vi "BusTapeAlignment.vi"() -> ()   [LabVIEW 2016]
uses:
  <vilib>/vision/Image Controls.llb/IMAQ Image.ctl
  <vilib>/vision/Measure.llb/Edge Options.ctl
  <vilib>/vision/Measure.llb/Edge Polarity.ctl
  <vilib>/Analysis/6fits.llb/Curve Fitting Criteria.ctl
  <vilib>/vision/NI_Vision_Development_Module.lvlib
  <vilib>/Analysis/NI_AALPro.lvlib
  <vilib>/Analysis/NI_AALBase.lvlib
panel:
  out "Image Frame":dbl[][](array[numeric])
  out "Locations":dbl[][](array[numeric])
  in  "Sample Size":dbl
  out "Output Cluster Array (Top/Bottom)":T1(array[cluster])
  in  "um/pix resolution":dbl=1.5
  in  "Template Path":path=path "D:/Git/StaveAssembly/XYZstage+Camera_CollectedImages/2017-03-03/1_Dots_WorkingDistanceCalibTemplate_z1p0.png"
  in  "Input Images Array":T2[](array[typedef])
  in  "Input Coordinate Array":dbl[][](array[numeric])
  in  "Test?":bool
  out "Bottom errors (um)":dbl[][](array[numeric])
  out "Top errors (um)":dbl[][](array[numeric])
  out "Bottom":cluster{"Bottom":dbl[], "Bottom":dbl[]}[](graph)
  out "Bottom \nResiduals (um)":dbl[](array[numeric])
  out "Top \nResiduals (um)":dbl[](array[numeric])
  out "Top":cluster{"Top":dbl[], "Top":dbl[]}[](graph)
  in  "method":T3 items=["Least Square", "Least Absolute Residual", "Bisquare"]
  out "Bottom":dbl[][](array[numeric])
  out "Top":dbl[][](array[numeric])
  out "Coordinate array for image capture":dbl[][](array[numeric])
  out "Processing Image #":i32
  out "Selected subarray":T2(plugin-control)
  out "Fitted Circle":T4 {"Average SNR (dB)" format="%.2f"; "Average Strength" format="%.2f"; "Roundness (Real-World)" format="%.2f"; "Radius (Real-World)" format="%.2f"; "Center (Real-World)"."Y" format="%.2f"; "Center (Real-World)"."X" format="%.2f"; "Radius (Pixels)" format="%.2f"; "Center (Pixels)"."Y" format="%.2f"; "Center (Pixels)"."X" format="%.2f"}
  in  "Circle ROI Descriptor":T5={"Global Rectangle"=[675, 567, 1751, 1642], "Contours"=[{"ID"=enum."External", "Type"=7, "Coordinates"=[1212, 1104, 190, 250, 0, 0]}]} {"Contours"."Type" items=["No Selection", "Point", "Line", "Rectangle", "Oval", "Polygon", "Freehand Region", "Annulus", "Unused2", "Unused3", "Broken Line", "Freehand Line", "Rotated Rectangle"]}
  in  "Circle Fit Options":T6={"Process"=enum."Get Best Edge", "Step Size"=3.0, "Max Pixel Radius"=3}
  in  "Circle Finding Options":T9={"Search  Direction"=1, "Edge Options"={"Edge Polarity"=2, "Kernel Size"=3, "Width"=3, "Minimum Edge Strength"=10.0, "Interpolation Type"=enum."Bilinear Fixed", "Data Processing Method"=enum."Median"}, "Show Search Area"=TRUE, "Show Search Lines"=TRUE, "Show Edges Found"=TRUE, "Show Result"=TRUE, "Search Area Color"=65280, "Search Lines Color"=255, "Edge Locations Color"=16776960, "Result Color"=65511, "Overlay Group Name"=""} {"Search  Direction" items=["Outside to Inside", "Inside to Outside"]; "Edge Options"."Edge Polarity" items=["All Edges", "Rising Edges", "Falling Edges"]; "Edge Options"."Minimum Edge Strength" format="%.2f"; "Edge Options"."Width" step=2; "Edge Options"."Kernel Size" step=2}
  in  "Pattern Match Settings":T10={"Algorithm"=2, "Number of Matches Requested"=1, "Minimum Match Score"=800.0, "SubPixel Accuracy"=TRUE, "Rotation Angle Ranges"=[], "Show Search Area"=FALSE, "Show Result"=TRUE} {"Rotation Angle Ranges"."End" format="%.1f"; "Rotation Angle Ranges"."Start" format="%.1f"; "Minimum Match Score" min=0 max=1000 format="%.2f"; "Number of Matches Requested" min=1; "Algorithm" items=["All", "Low Discrepancy Sampling", "Grayscale Value Pyramid", "Gradients Pyramid"]}
  out "Template Image":T2
  in  "Coordinate file for image capture":path=path "D:/Git/StaveAssembly/XYZstage+Camera_CollectedImages/2017-03-15/BrendonsFidMarks_dots_2017-03-15-captured.csv"
  out "Review":bool
  out "Search running?":bool
  in  "Stop and delete":bool
  out "Images Array":T2[](array[plugin-control])=["image_442_-22_00"]
  in  "error in":errorcluster
  out "error out":errorcluster
  out "Filenames Array":string[](array[string])=["image_442_-22_110.png", "image_442_-22_137.png", "image_442_-22_192.png", "image_442_-22_222.png", "image_442_-22_26.png", "image_442_-22_56.png"]
  in  "Naming Convention":string="image_*_*_*_*.png"
  in  "Images Directory":path=path "D:/Git/StaveAssembly/XYZstage+Camera_CollectedImages/2017-03-15/images"
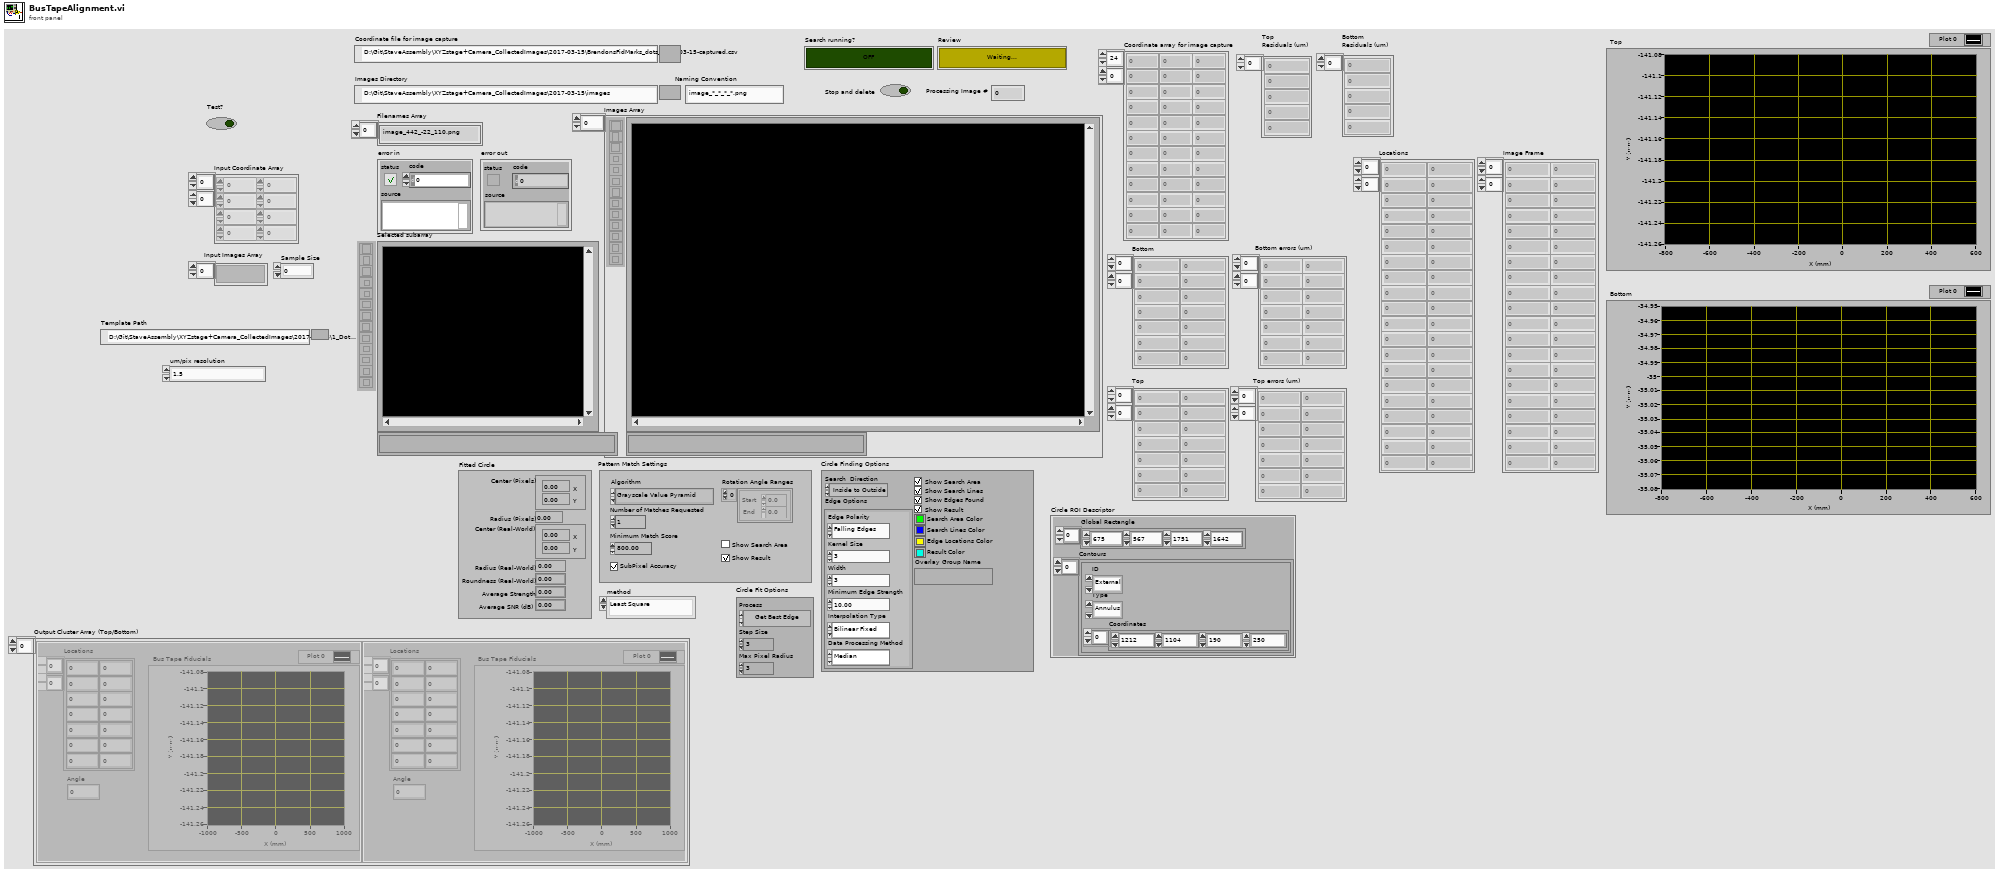
[diagram p1: front panel]
types:
  T1 = cluster{"Locations":dbl[][], "Angle":dbl, "Bus Tape Fiducials":cluster{"Bottom":dbl[], "Bottom":dbl[]}[]}[]
  T2 = typedef "IMAQ Image.ctl" = refnum<image>
  T3 = typedef "NI_AALPro.lvlib/Curve Fitting Criteria.ctl" = u16
  T4 = cluster{"Center (Pixels)":cluster{"X":sgl, "Y":sgl}, "Radius (Pixels)":dbl, "Center (Real-World)":cluster{"X":sgl, "Y":sgl}, "Radius (Real-World)":dbl, "Roundness (Real-World)":dbl, "Average Strength":dbl, "Average SNR (dB)":dbl}
  T5 = cluster{"Global Rectangle":i32[], "Contours":cluster{"ID":enum32{"External", "Internal"}, "Type":u32, "Coordinates":i32[]}[]}
  T6 = cluster{"Process":enum16{"Get First Edge", "Get First + Last Edge", "Get All Edges", "Get Best Edge"}, "Step Size":dbl, "Max Pixel Radius":i32}
  T7 = typedef "Edge Options.ctl" = cluster{"Edge Polarity":T8, "Kernel Size":u32, "Width":u32, "Minimum Edge Strength":sgl, "Interpolation Type":enum32{"Zero Order", "Bilinear", "Quadratic", "Cubic", "Bilinear Fixed"}, "Data Processing Method":enum32{"Average", "Median"}}
  T8 = typedef "Edge Polarity.ctl" = u32
  T9 = cluster{"Search  Direction":u32, "Edge Options":T7, "Show Search Area":bool, "Show Search Lines":bool, "Show Edges Found":bool, "Show Result":bool, "Search Area Color":u32, "Search Lines Color":u32, "Edge Locations Color":u32, "Result Color":u32, "Overlay Group Name":string}
  T10 = cluster{"Algorithm":i32, "Number of Matches Requested":i32, "Minimum Match Score":sgl, "SubPixel Accuracy":bool, "Rotation Angle Ranges":cluster{"Start":sgl, "End":sgl}[], "Show Search Area":bool, "Show Result":bool}
  T11 = cluster{"Position":cluster{"x":sgl, "y":sgl}, "Angle":sgl, "Scale":sgl, "Score":sgl, "Bounding Box":cluster{"x":sgl, "y":sgl}[]}[]
  T12 = cluster{"Global Rectangle":i32[], cluster{"ID":enum32{"External", "Internal"}, "Type":u32, "Coordinates":i32[]}[]}
  T13 = cluster{"Top":dbl[][], dbl, cluster{"Top":dbl[], "Top":dbl[]}[]}
  T14 = cluster{"Bottom":dbl[][], dbl, cluster{"Bottom":dbl[], "Bottom":dbl[]}[]}
  T15 = cluster{"Bottom":dbl[][], dbl, cluster{"Bottom":dbl[], "Bottom":dbl[]}[]}[]
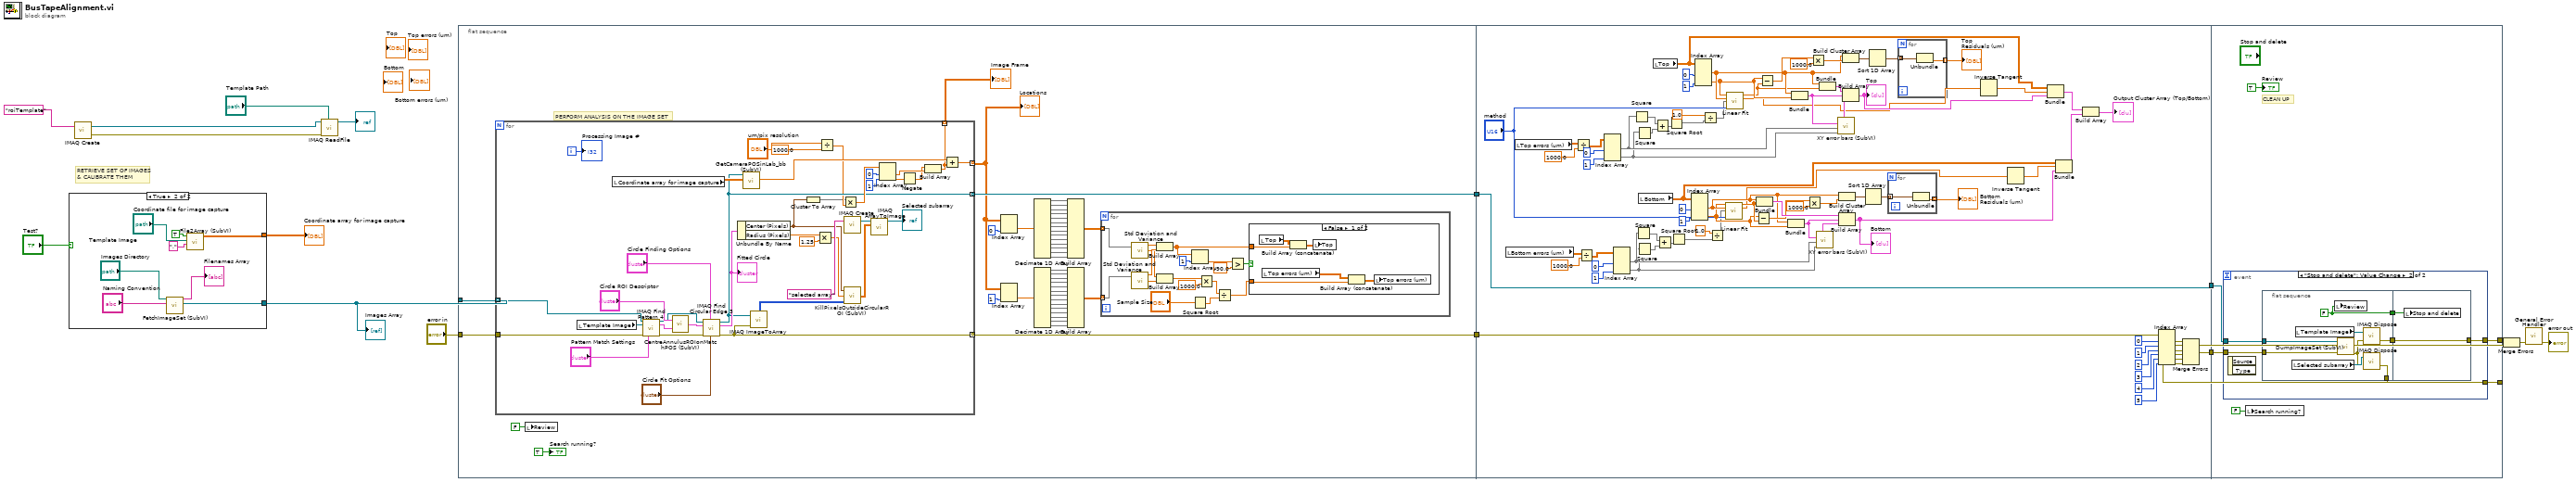
[diagram p0: block diagram]
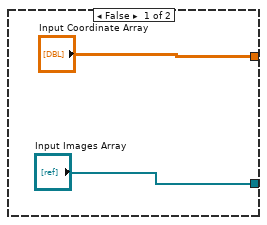
[diagram p2: hidden frame]
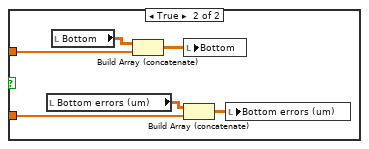
[diagram p3: hidden frame]
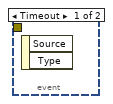
[diagram p4: hidden frame]
diagram:
  # "RETRIEVE SET OF IMAGES\n& CALIBRATE THEM"
  n1 = case shown="True" "Test?" {
    tunnel: ["Input Coordinate Array" w24] -> w4
    tunnel: ["Input Images Array" w20] -> w2
    frame False {
    }
    frame True {
      n2 = call "FetchImageSet (SubVI).vi"("Naming Convention"="Naming Convention", "Images Directory"="Images Directory") -> ("Image Array"=w20:T2[], "Filenames Array"=→"Filenames Array":string[])  [unwired: 7 in, 1 out]
      n3 = call "File2Array (SubVI).vi"("File delimiter"=",", "Source array file"="Coordinate file for image capture", "Load array from file?"=TRUE) -> ("Loaded array"=w24:dbl[][])  [unwired: 7 in, 1 out]
    }
  }
  "Coordinate array for image capture" <- w4
  "Images Array" <- w2
  n4 = call "IMAQ Create"("Image Name"="roiTemplate") -> ("New Image"=w7:T2, "error out"=w13:errorcluster)  [unwired: 4 in]
  n5 = call "IMAQ ReadFile"("File Path"="Template Path", "error in (no error)"=w13, "Image"=w7) -> ("Image Out"=→"Template Image":T2)  [unwired: 4 in, 4 out]
  n6 = flat-sequence {
    tunnel: w2 -> [w67]
    tunnel: "error in" -> [w66]
    tunnel: [w65] -> w10
    tunnel: [w64] -> w9
    tunnel: [w217] -> w12
    tunnel: w10 -> [w217]
    tunnel: w9 -> [w215]
    tunnel: [w216] -> w8
    tunnel: [w225] -> w16
    tunnel: w12 -> [w224]
    tunnel: [w223] -> w11
    tunnel: w8 -> [w222]
    frame #0 {
      # "PERFORM ANALYSIS ON THE IMAGE SET"
      n7 = for {
        tunnel: w67 -> [w136] mode=indexing
        tunnel: w66 -> [w134]
        tunnel: [w113] -> w65 mode=indexing
        tunnel: [w117] -> w64 mode=indexing
        tunnel: [w101] -> w29 mode=indexing
        tunnel: [w99] -> w28 mode=indexing
        i -> [w105]
        n8 = local read "Template Image"() -> (w115:T2)
        n9 = local read "Coordinate array for image capture"() -> (w114:dbl[][])
        n10 = call "IMAQ Find Pattern 4"("Image"=w136, "Template"=w115, "error in"=w134, "Settings"="Pattern Match Settings") -> ("Image Out"=w109:T2, "Matches (pixel)"=w131:T11, "error out"=w107:errorcluster)  [unwired: 5 in, 4 out]
        n11 = call "CentreAnnulusROIonMatchPOS (SubVI).vi"("Matches (pixel)"=w131, "Annulus ROI Descriptor"="Circle ROI Descriptor") -> ("Annulus ROI Descriptor centred on match position"=w108:T12)
        n12 = call "IMAQ Find Circular Edge 3"("Circle Fit Options"="Circle Fit Options", "Options"="Circle Finding Options", "error in (no error)"=w107, "ROI Descriptor"=w108, "Image"=w109) -> ("error out"=w117:errorcluster, "Fitted Circle"=w125:T4, "Image Out"=w113:T2)  [unwired: 2 in, 2 out]
        "Fitted Circle" <- w125
        n13 = Unbundle By Name(w125) -> ("Center (Pixels)"=w124:cluster{"X":sgl, "Y":sgl}, "Radius (Pixels)"=w116:dbl)
        n14 = call "GetCameraPOSinLab_bb (SubVI).vi"("Loaded array"=w114, "Refnum in"=w113) -> ("Image coordinates in lab frame"=w106:dbl[])  [unwired: 7 in, 2 out]
        n15 = call "IMAQ ImageToArray"("error in (no error)"=w117, "Image"=w113) -> ("Image Pixels (U8)"=w129:u8[][])  [unwired: 2 in, 4 out]
        n16 = Cluster To Array(cluster=w124) -> (array=w100:sgl[])
        n17 = Multiply(x=w116, y=1.25) -> (x*y=w111:dbl)
        n18 = Divide(x="um/pix resolution", y=1000.0) -> (x/y=w102:dbl)
        n19 = Multiply(x=w100, y=w102) -> (x*y=w123:dbl[])
        n20 = call "IMAQ Create"("Image Name"="selected array") -> ("New Image"=w127:T2)  [unwired: 4 in, 1 out]
        n21 = call "KillPixelsOutsideCircularROI (SubVI).vi"("XY Array"=w129, "Radius*ScaleFactor"=w111, "Center (Pixels)"=w124) -> ("subarray"=w112:dbl[][])
        n22 = call "IMAQ ArrayToImage"("Image Pixels (U8)"=w112, "Image"=w127) -> ("Image Out"=→"Selected subarray":T2)  [unwired: 8 in, 1 out]
        n23 = Index Array(array=w123, index #1=0, index #2=1) -> (element #1=w119:dbl, element #2=w120:dbl)
        n24 = Negate(x=w120) -> (-x=w118:dbl)
        n25 = Build Array(w118, w119) -> (w99:dbl[])
        n26 = Add(x=w106, y=w99) -> (x+y=w101:dbl[])
        "Processing Image #" <- w105
      }
      "Locations" <- w29
      "Image Frame" <- w28
      n27 = local write "Review"(FALSE ("Review")) -> ()
      n28 = Index Array(array=w29, index (col)=0) -> (element=w31:dbl[])  [unwired: 1 in]
      n29 = Index Array(array=w29, index (col)=1) -> (element=w30:dbl[])  [unwired: 1 in]
      n30 = Decimate 1D Array(w31) -> (w61:dbl[], w60:dbl[], w59:dbl[], w58:dbl[], w57:dbl[], w56:dbl[], w55:dbl[], w54:dbl[], w53:dbl[], w52:dbl[], w51:dbl[], w50:dbl[], w49:dbl[], w48:dbl[])
      n31 = Decimate 1D Array(w30) -> (w47:dbl[], w46:dbl[], w45:dbl[], w44:dbl[], w43:dbl[], w42:dbl[], w41:dbl[], w40:dbl[], w39:dbl[], w38:dbl[], w37:dbl[], w36:dbl[], w35:dbl[], w34:dbl[])
      n32 = Build Array(w61, w60, w59, w58, w57, w56, w55, w54, w53, w52, w51, w50, w49, w48) -> (w33:dbl[][])
      n33 = Build Array(w47, w46, w45, w44, w43, w42, w41, w40, w39, w38, w37, w36, w35, w34) -> (w32:dbl[][])
      n34 = for {
        tunnel: w33 -> [w86] mode=indexing
        tunnel: w32 -> [w85] mode=indexing
        n35 = call <vilib>:"Std Deviation and Variance.vi"("X"=w86) -> ("mean"=w84:dbl, "standard deviation"=w82:dbl)  [unwired: 1 in, 1 out]
        n36 = call <vilib>:"Std Deviation and Variance.vi"("X"=w85) -> ("mean"=w83:dbl, "standard deviation"=w81:dbl)  [unwired: 1 in, 1 out]
        n37 = Build Array(w84, w83) -> (w74:dbl[])
        n38 = Build Array(w82, w81) -> (w80:dbl[])
        n39 = Index Array(array=w74, index=1) -> (element=w76:dbl)
        n40 = Square Root(x="Sample Size") -> (sqrt(x)=w72:dbl)
        n41 = Multiply(x=w80, y=1000.0) -> (x*y=w71:dbl[])
        n42 = Divide(x=w71, y=w72) -> (x/y=w70:dbl[])
        n43 = Greater?(x=w76, y=-90.0) -> (0:w78:bool)
        n44 = case shown="False" w78 {
          tunnel: w74 -> [w90 w97]
          tunnel: w70 -> [w88 w93]
          frame False {
            n45 = local read "Top"() -> (w92:dbl[][])
            n46 = local read "Top errors (um)"() -> (w87:dbl[][])
            n47 = Build Array (concatenate)(w92, w90) -> (w91:dbl[][])
            n48 = local write "Top"(w91) -> ()
            n49 = Build Array (concatenate)(w87, w88) -> (w89:dbl[][])
            n50 = local write "Top errors (um)"(w89) -> ()
          }
          frame True {
            n51 = local read "Bottom errors (um)"() -> (w94:dbl[][])
            n52 = local read "Bottom"() -> (w98:dbl[][])
            n53 = Build Array (concatenate)(w98, w97) -> (w96:dbl[][])
            n54 = local write "Bottom"(w96) -> ()
            n55 = Build Array (concatenate)(w94, w93) -> (w95:dbl[][])
            n56 = local write "Bottom errors (um)"(w95) -> ()
          }
        }
      }
      "Search running?" <- TRUE ("Search running?")
    }
    frame #1 {
      n57 = local read "Bottom errors (um)"() -> (w172:dbl[][])
      n58 = local read "Top errors (um)"() -> (w173:dbl[][])
      n59 = Divide(x=w173, y=1000.0) -> (x/y=w163:dbl[][])
      n60 = Divide(x=w172, y=1000.0) -> (x/y=w168:dbl[][])
      n61 = Index Array(array=w163, index (col) #1=0, index (col) #2=1) -> (element #1=w162:dbl[], element #2=w156:dbl[])  [unwired: 2 in]
      n62 = Index Array(array=w168, index (col) #1=0, index (col) #2=1) -> (element #1=w151:dbl[], element #2=w150:dbl[])  [unwired: 2 in]
      n63 = Square(x=w162) -> (x^2=w159:dbl[])
      n64 = Square(x=w151) -> (x^2=w155:dbl[])
      n65 = Square(x=w156) -> (x^2=w157:dbl[])
      n66 = Square(x=w150) -> (x^2=w153:dbl[])
      n67 = local read "Bottom"() -> (w141:dbl[][])
      n68 = local read "Top"() -> (w147:dbl[][])
      n69 = Add(x=w159, y=w157) -> (x+y=w158:dbl[])
      n70 = Add(x=w155, y=w153) -> (x+y=w154:dbl[])
      n71 = Square Root(x=w158) -> (sqrt(x)=w160:dbl[])
      n72 = Square Root(x=w154) -> (sqrt(x)=w149:dbl[])
      n73 = Index Array(array=w141, index (col) #1=0, index (col) #2=1) -> (element #1=w190:dbl[], element #2=w180:dbl[])  [unwired: 2 in]
      n74 = Index Array(array=w147, index (col) #1=0, index (col) #2=1) -> (element #1=w184:dbl[], element #2=w179:dbl[])  [unwired: 2 in]
      n75 = Divide(x=1.0, y=w160) -> (x/y=w161:dbl[])
      n76 = Divide(x=1.0, y=w149) -> (x/y=w152:dbl[])
      n77 = call <vilib>:"Linear Fit.vi"("Y"=w180, "X"=w190, "Weight"=w152, "method"="method") -> ("Best Linear Fit"=w181:dbl[], "slope"=w142:dbl)  [unwired: 7 in, 3 out]
      n78 = call <vilib>:"Linear Fit.vi"("Y"=w179, "X"=w184, "Weight"=w161, "method"="method") -> ("Best Linear Fit"=w148:dbl[], "slope"=w143:dbl)  [unwired: 7 in, 3 out]
      n79 = Subtract(x=w180, y=w181) -> (x-y=w194:dbl[])
      n80 = Bundle("Bottom"=w190, "Best Linear Fit"=w181) -> (w195:cluster{"Bottom":dbl[], "Best Linear Fit":dbl[]})  [unwired: 1 in]
      n81 = Subtract(x=w179, y=w148) -> (x-y=w199:dbl[])
      n82 = Bundle("Bottom"=w190, "Bottom"=w180) -> (w178:cluster{"Bottom":dbl[], "Bottom":dbl[]})  [unwired: 1 in]
      n83 = Bundle("Top"=w184, "Top"=w179) -> (w175:cluster{"Top":dbl[], "Top":dbl[]})  [unwired: 1 in]
      n84 = Multiply(x=w194, y=1000.0) -> (x*y=w191:dbl[])
      n85 = Multiply(x=w199, y=1000.0) -> (x*y=w186:dbl[])
      n86 = call "XY error bars (SubVI).vi"("XY plot"=w178, "Xerror"=w151, "Yerror"=w150) -> ("X+Y error bars"=w169:cluster{dbl[], dbl[]})  [unwired: 5 in, 2 out]
      n87 = Bundle("Top"=w184, "Best Linear Fit"=w148) -> (w200:cluster{"Top":dbl[], "Best Linear Fit":dbl[]})  [unwired: 1 in]
      n88 = call "XY error bars (SubVI).vi"("XY plot"=w175, "Xerror"=w162, "Yerror"=w156) -> ("X+Y error bars"=w170:cluster{dbl[], dbl[]})  [unwired: 5 in, 2 out]
      n89 = Build Cluster Array(w190, w191) -> (w189:cluster{"Numeric":dbl, dbl}[])
      n90 = Build Array(w195, w178, w169) -> (w140:cluster{"Bottom":dbl[], "Bottom":dbl[]}[])
      "Bottom" <- w140
      n91 = Build Cluster Array(w184, w186) -> (w185:cluster{"Numeric":dbl, dbl}[])
      n92 = Build Array(w200, w175, w170) -> (w145:cluster{"Top":dbl[], "Top":dbl[]}[])
      "Top" <- w145
      n93 = Sort 1D Array(array=w189) -> (sorted array=w188:cluster{"Numeric":dbl, dbl}[])
      n94 = Sort 1D Array(array=w185) -> (sorted array=w183:cluster{"Numeric":dbl, dbl}[])
      n95 = for {
        tunnel: w188 -> [w221] mode=indexing
        tunnel: [w220] -> w187 mode=indexing
        n96 = Unbundle(w221) -> (w220:dbl)  [unwired: 1 out]
      }
      "Bottom \nResiduals (um)" <- w187
      n97 = for {
        tunnel: w183 -> [w219] mode=indexing
        tunnel: [w218] -> w182 mode=indexing
        n98 = Unbundle(w219) -> (w218:dbl)  [unwired: 1 out]
      }
      "Top \nResiduals (um)" <- w182
      n99 = Inverse Tangent(1:w143) -> (0:w146:dbl)
      n100 = Inverse Tangent(1:w142) -> (0:w144:dbl)
      n101 = Bundle("Top"=w147, w146, w145) -> (w139:T13)  [unwired: 1 in]
      n102 = Bundle("Bottom"=w141, w144, w140) -> (w138:T14)  [unwired: 1 in]
      n103 = Build Array(w139, w138) -> (→"Output Cluster Array (Top/Bottom)":T15)
      n104 = Index Array(array=w215, index #1=0, index #2=1, index #3=2, index #4=3, index #5=4, index #6=5) -> (element #1=w214:errorcluster, element #2=w213:errorcluster, element #3=w212:errorcluster, element #4=w211:errorcluster, element #5=w210:errorcluster, element #6=w209:errorcluster)
      n105 = Merge Errors(w214, w213, w212, w211, w210, w209) -> (w216:errorcluster)
    }
    frame #2 {
      # "CLEAN UP"
      n106 = event shown="[1] \"Stop and delete\": Value Change" {
        selector: _ -> [_ _]
        dyn-events: _ -> [_ _]
        timeout: _ -> [_ _]
        tunnel: [_ w233] -> w225
        tunnel: w224 -> [_ w230]
        tunnel: [_ w229] -> w223
        tunnel: w222 -> [_ w228]
        event Timeout {
          n107 = event-data() -> ()  [unwired: 1 in, 2 out]
        }
        event "Stop and delete": Value Change {
          n108 = event-data() -> ()  [unwired: 1 in, 2 out]
          n109 = flat-sequence {
            tunnel: [w240] -> w232
            tunnel: [w239] -> w231
            tunnel: w230 -> [w238]
            tunnel: w228 -> [w234]
            tunnel: [w235] -> w229
            tunnel: [w243] -> w233
            tunnel: w232 -> [w243]
            tunnel: w231 -> [w242]
            frame #0 {
              w239 = FALSE ("Review")
              n110 = local read "Selected subarray"() -> (w237:T2)
              n111 = local read "Template Image"() -> (w241:T2)
              n112 = local write "Review"(w239) -> ()
              n113 = call "DumpImageSet (SubVI).vi"("error in (no error)"=w234, "Calibrated Image Array"=w238) -> ("error out"=w236:errorcluster)  [unwired: 6 in]
              n114 = call "IMAQ Dispose"("Image"=w241, "error in (no error)"=w236) -> ("error out"=w240:errorcluster)  [unwired: 4 in]
              n115 = call "IMAQ Dispose"("Image"=w237, "error in (no error)"=w236) -> ("error out"=w235:errorcluster)  [unwired: 4 in]
            }
            frame #1 {
              n116 = local write "Stop and delete"(w242) -> ()
            }
          }
        }
      }
      n117 = local write "Search running?"(FALSE ("Search running?")) -> ()
      "Review" <- TRUE ("Review")
    }
  }
  n118 = Merge Errors(w16, w11) -> (w15:errorcluster)
  n119 = call <vilib>:"General Error Handler.vi"("error in (no error)"=w15) -> ("error out"=→"error out":errorcluster)  [unwired: 10 in, 4 out]
